vi "Player Info.vi"(8 "Victory Speech":string="You just got spwned!", 9 "Name":string="Spawn", 11 "Spawn in":refnum<class "Spawn.lvclass">) -> (3 "Spawn out":refnum<class "Spawn.lvclass">)   [LabVIEW 2015, in "Spawn.lvclass"]
uses:
  Spawn.lvclass
  Square/Square.lvclass
panel:
  # "Set default values for these two string controls"
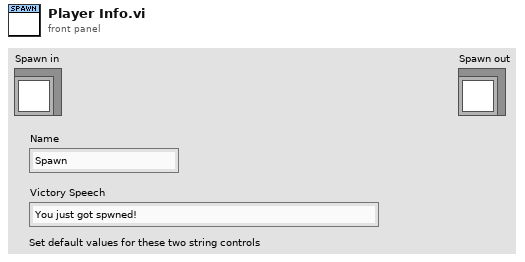
[diagram p1: front panel]
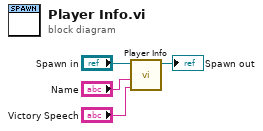
[diagram p0: block diagram]
diagram:
  n1 = call-parent "Player Info.vi"("Victory Speech"="Victory Speech", "Name"="Name", "Square in"="Spawn in") -> ("Square out"=→"Spawn out":refnum<class "Spawn.lvclass">)  [unwired: 8 in]
